vi "KB-sub求波形的前后最高点.vi"(11 "中间行波形":dbl[](graph)) -> (0 "后半部分高度平均值":dbl, 3 "前半部分高度平均值":dbl)   [LabVIEW 2015]
panel:
  out "后半部分波形":dbl[](graph)
  out "前半部分波形":dbl[](graph)
  out "x/y":dbl
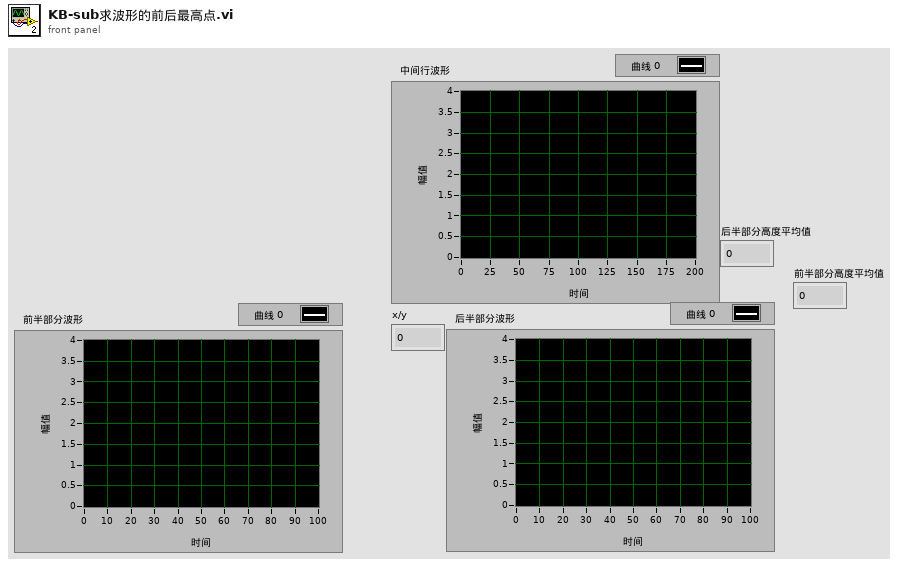
[diagram p1: front panel]
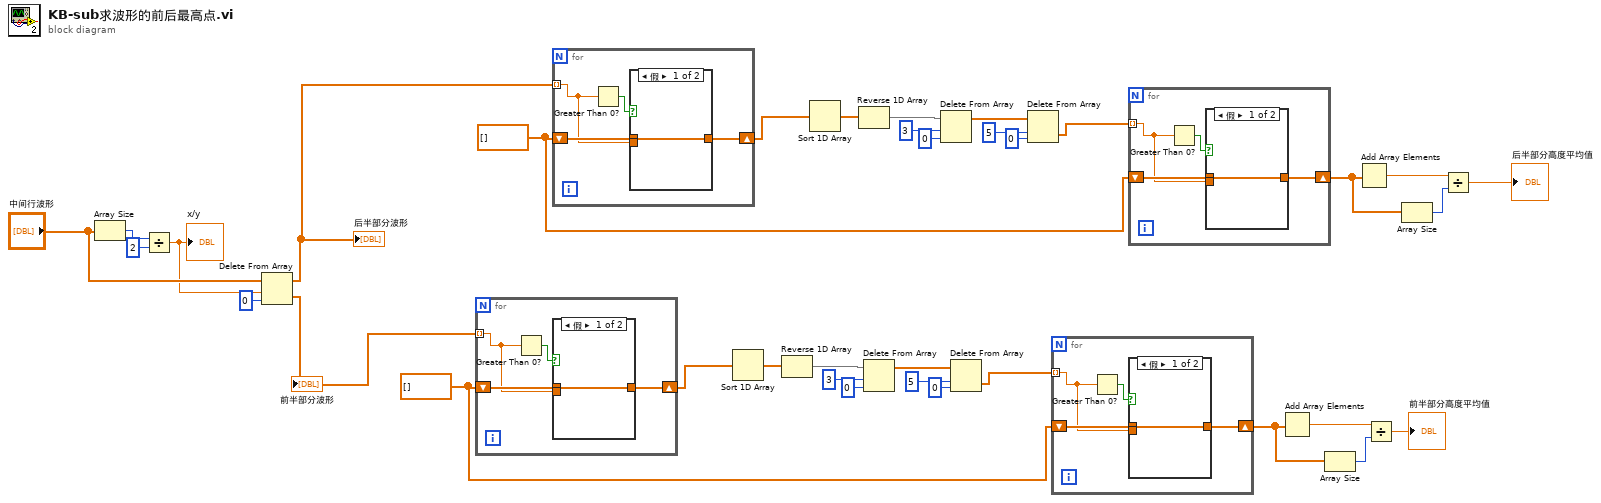
[diagram p0: block diagram]
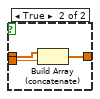
[diagram p2: hidden frame]
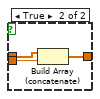
[diagram p3: hidden frame]
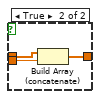
[diagram p4: hidden frame]
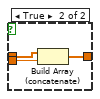
[diagram p5: hidden frame]
diagram:
  w11 = dbl[] []
  w21 = dbl[] []
  n1 = Array Size(array="中间行波形") -> (size(s)=w35:i32)
  n2 = Divide(x=w35, y=2) -> (x/y=w31:dbl)
  "x/y" <- w31
  n3 = Delete From Array(array="中间行波形", length=w31, index=0 ("索引")) -> (deleted portion=w30:dbl[], array with subset deleted=w2:dbl[])
  "前半部分波形" <- w30
  "后半部分波形" <- w2
  n4 = for {
    tunnel: w30 -> [w37] mode=indexing
    shift-right: [w36] -> w29
    shift-left: w21 -> [w38]
    n5 = Greater Than 0?(x=w37) -> (x > 0?=w39:bool)
    n6 = case shown="假" w39 {
      tunnel: w38 -> [w40 w43]
      tunnel: w37 -> [_ w42]
      tunnel: [w40 w41] -> w36
      frame False {
      }
      frame True {
        n7 = Build Array (concatenate)(w43, w42) -> (w41:dbl[])
      }
    }
  }
  n8 = for {
    tunnel: w2 -> [w45] mode=indexing
    shift-right: [w44] -> w3
    shift-left: w11 -> [w46]
    n9 = Greater Than 0?(x=w45) -> (x > 0?=w47:bool)
    n10 = case shown="假" w47 {
      tunnel: w46 -> [w48 w51]
      tunnel: w45 -> [_ w50]
      tunnel: [w48 w49] -> w44
      frame False {
      }
      frame True {
        n11 = Build Array (concatenate)(w51, w50) -> (w49:dbl[])
      }
    }
  }
  n12 = Sort 1D Array(array=w29) -> (sorted array=w28:dbl[])
  n13 = Reverse 1D Array(array=w28) -> (reversed array=w27:dbl[])
  n14 = Sort 1D Array(array=w3) -> (sorted array=w4:dbl[])
  n15 = Reverse 1D Array(array=w4) -> (reversed array=w5:dbl[])
  n16 = Delete From Array(array=w27, length=3 ("长度"), index=0 ("索引")) -> (array with subset deleted=w22:dbl[])  [unwired: 1 out]
  n17 = Delete From Array(array=w5, length=3 ("长度"), index=0 ("索引")) -> (array with subset deleted=w10:dbl[])  [unwired: 1 out]
  n18 = Delete From Array(array=w22, length=5 ("长度"), index=0 ("索引")) -> (deleted portion=w16:dbl[])  [unwired: 1 out]
  n19 = Delete From Array(array=w10, length=5 ("长度"), index=0 ("索引")) -> (deleted portion=w15:dbl[])  [unwired: 1 out]
  n20 = for {
    tunnel: w16 -> [w53] mode=indexing
    shift-right: [w52] -> w17
    shift-left: w21 -> [w54]
    n21 = Greater Than 0?(x=w53) -> (x > 0?=w55:bool)
    n22 = case shown="假" w55 {
      tunnel: w54 -> [w56 w59]
      tunnel: w53 -> [_ w58]
      tunnel: [w56 w57] -> w52
      frame False {
      }
      frame True {
        n23 = Build Array (concatenate)(w59, w58) -> (w57:dbl[])
      }
    }
  }
  n24 = for {
    tunnel: w15 -> [w61] mode=indexing
    shift-right: [w60] -> w14
    shift-left: w11 -> [w62]
    n25 = Greater Than 0?(x=w61) -> (x > 0?=w63:bool)
    n26 = case shown="假" w63 {
      tunnel: w62 -> [w64 w67]
      tunnel: w61 -> [_ w66]
      tunnel: [w64 w65] -> w60
      frame False {
      }
      frame True {
        n27 = Build Array (concatenate)(w67, w66) -> (w65:dbl[])
      }
    }
  }
  n28 = Add Array Elements(numeric array=w17) -> (sum=w20:dbl)
  n29 = Array Size(array=w17) -> (size(s)=w19:i32)
  n30 = Add Array Elements(numeric array=w14) -> (sum=w12:dbl)
  n31 = Divide(x=w20, y=w19) -> (x/y=→"前半部分高度平均值":dbl)
  n32 = Array Size(array=w14) -> (size(s)=w13:i32)
  n33 = Divide(x=w12, y=w13) -> (x/y=→"后半部分高度平均值":dbl)
